vi "velocity control.vi"() -> ()   [LabVIEW 2018]
uses:
  <vilib>/Platform/TimedLoop/XDataNode/timing_clust.ctl
  <vilib>/Platform/TimedLoop/XDataNode/nitl_modes.ctl
  <vilib>/Platform/TimedLoop/XDataNode/wakeup.ctl
  <vilib>/FPGAPlugInAG/myRIO-1900/niLvFpga_Open_myRIO-1900.vi
  <vilib>/rvi/interface/common/dynamic/niFpgaDynamicAddResources.vi
  <vilib>/Utility/error.llb/Error Cluster From Error Code.vi
  <vilib>/rvi/errors/niLvFpgaAdjustHostInterfaceError.vi
  <vilib>/rvi/interface/nirviOpenFPGA/nirviOpenFPGA.xnode
  FPGA Bitfiles/Dentalrobot_FPGATarget_FPGADentalroboto_PTkoih3chUc.lvbitx
  FPGA/FPGA_myRIO.vi
  <vilib>/rvi/interface/nirviReadWriteControl/nirviReadWriteControl.xnode
  <vilib>/Platform/TimedLoop/XDataNode/XDataNode.xnode
  <vilib>/Platform/TimedLoop/XDataNode/XDNodeRunTimeDep.lvlib
  <vilib>/rvi/interface/Simulation/niFpgaSimulationCallBeginRW.vi
  NiFpgaLv.dll
panel:
  out "V' 2":dbl
  out "Waveform Chart 2":dbl(graph)
  out "Duty Cycle (Abs)":dbl
  in  "PID Gains":cluster{"Kp":dbl, "Kd":dbl, "Ki":dbl}={"Kp"=0.0021, "Kd"=0.0005, "Ki"=0.0005} {"Kp" step=0.001 format="%#_8f"; "Kd" step=0.01; "Ki" format="%#_6f"}
  out "V'":dbl
  in  "Desired Velocity":dbl step=10.0
  in  "Counts/revolution":i32=34304
  out "JumpBy2Error 4":i16
  out "Waveform Chart":dbl(graph)
  in  "stop":bool
  out "Position4":i32
  in  "Reset 4":bool
  in  "DIR4":bool
  in  "ENA4":bool
  out "finished late":dbl
  # "275:1   140800\n67:1      34304"
  # "rpm"
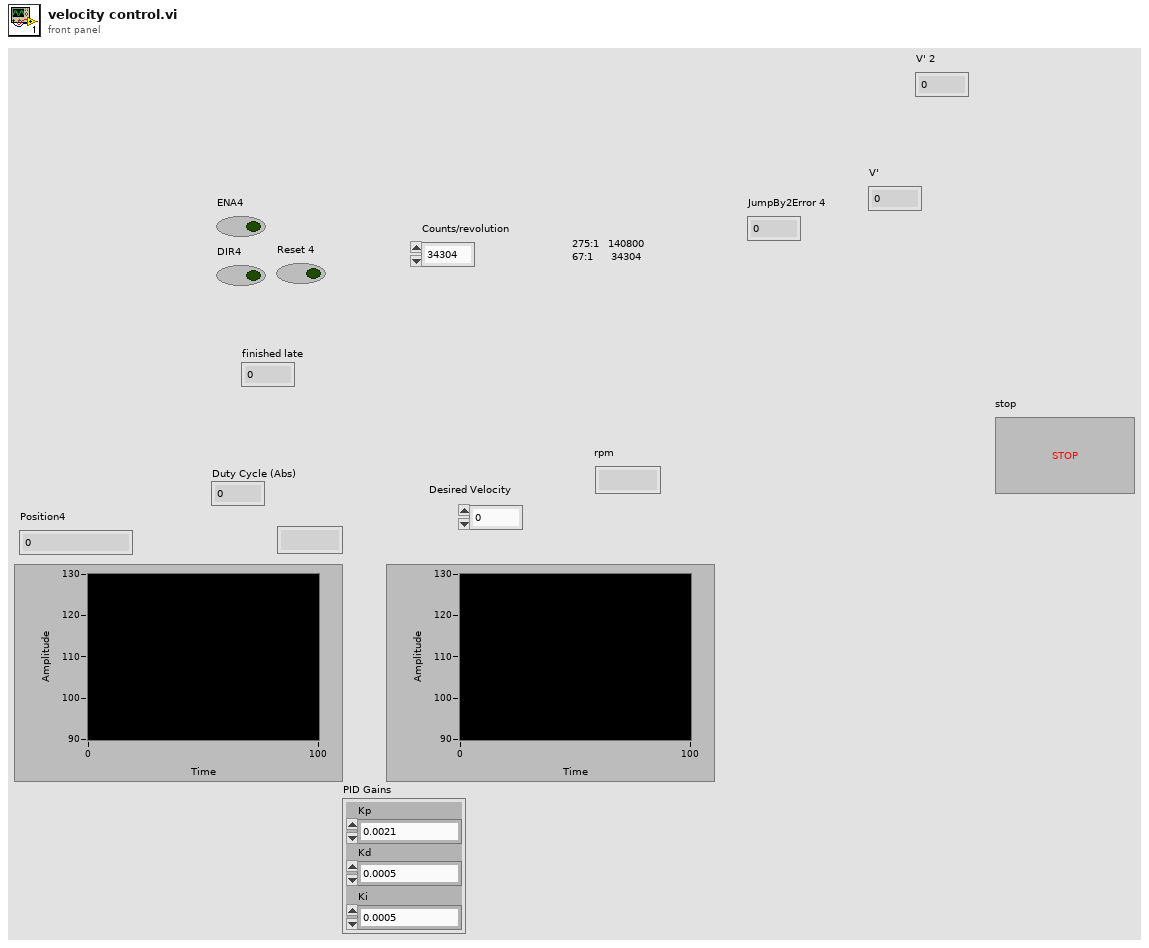
[diagram p1: front panel]
types:
  T1 = typedef "XDNodeRunTimeDep.lvlib/timing_clust.ctl" = cluster{"Expected End [f-1]":u64, "Actual End [f-1]":u64, "Finished Late? [f-1]":bool, "Expected End [i-1]":u64, "Actual End [i-1]":u64, "Finished Late? [i-1]":bool, "Expected Start [i]":u64, "Actual Start [i]":u64, "Expected Start [f]":u64, "Actual Start [f]":u64, "Source Name":string, "Structure Name":string, "Period":i64, "Deadline":i64, "Offset":i64, "Start":i64, "Priority":i32, "Timeout":i32, "Mode":T2, "Wakeup Reason":T3, "Error":errorcluster, "Source Type":string, "Secondary Source Type":string, "Global End Time":u64, "Global Start Time":u64, "Frame Duration":u64, "Iteration Duration":u64, "Assigned CPU":i32, "I/O Scan Engine Mode":u32}
  T2 = typedef "XDNodeRunTimeDep.lvlib/nitl_modes.ctl" = enum32{"No Change", "Process missed periods, maintain original phase", "Discard missed periods, maintain original phase", "Process missed periods, ignore original phase", "Discard missed periods, ignore original phase"}
  T3 = typedef "XDNodeRunTimeDep.lvlib/wakeup.ctl" = enum32{"Normal", "Aborted", "Asynchronous wakeup", "Timing source error", "Timed loop error", "Timeout"}
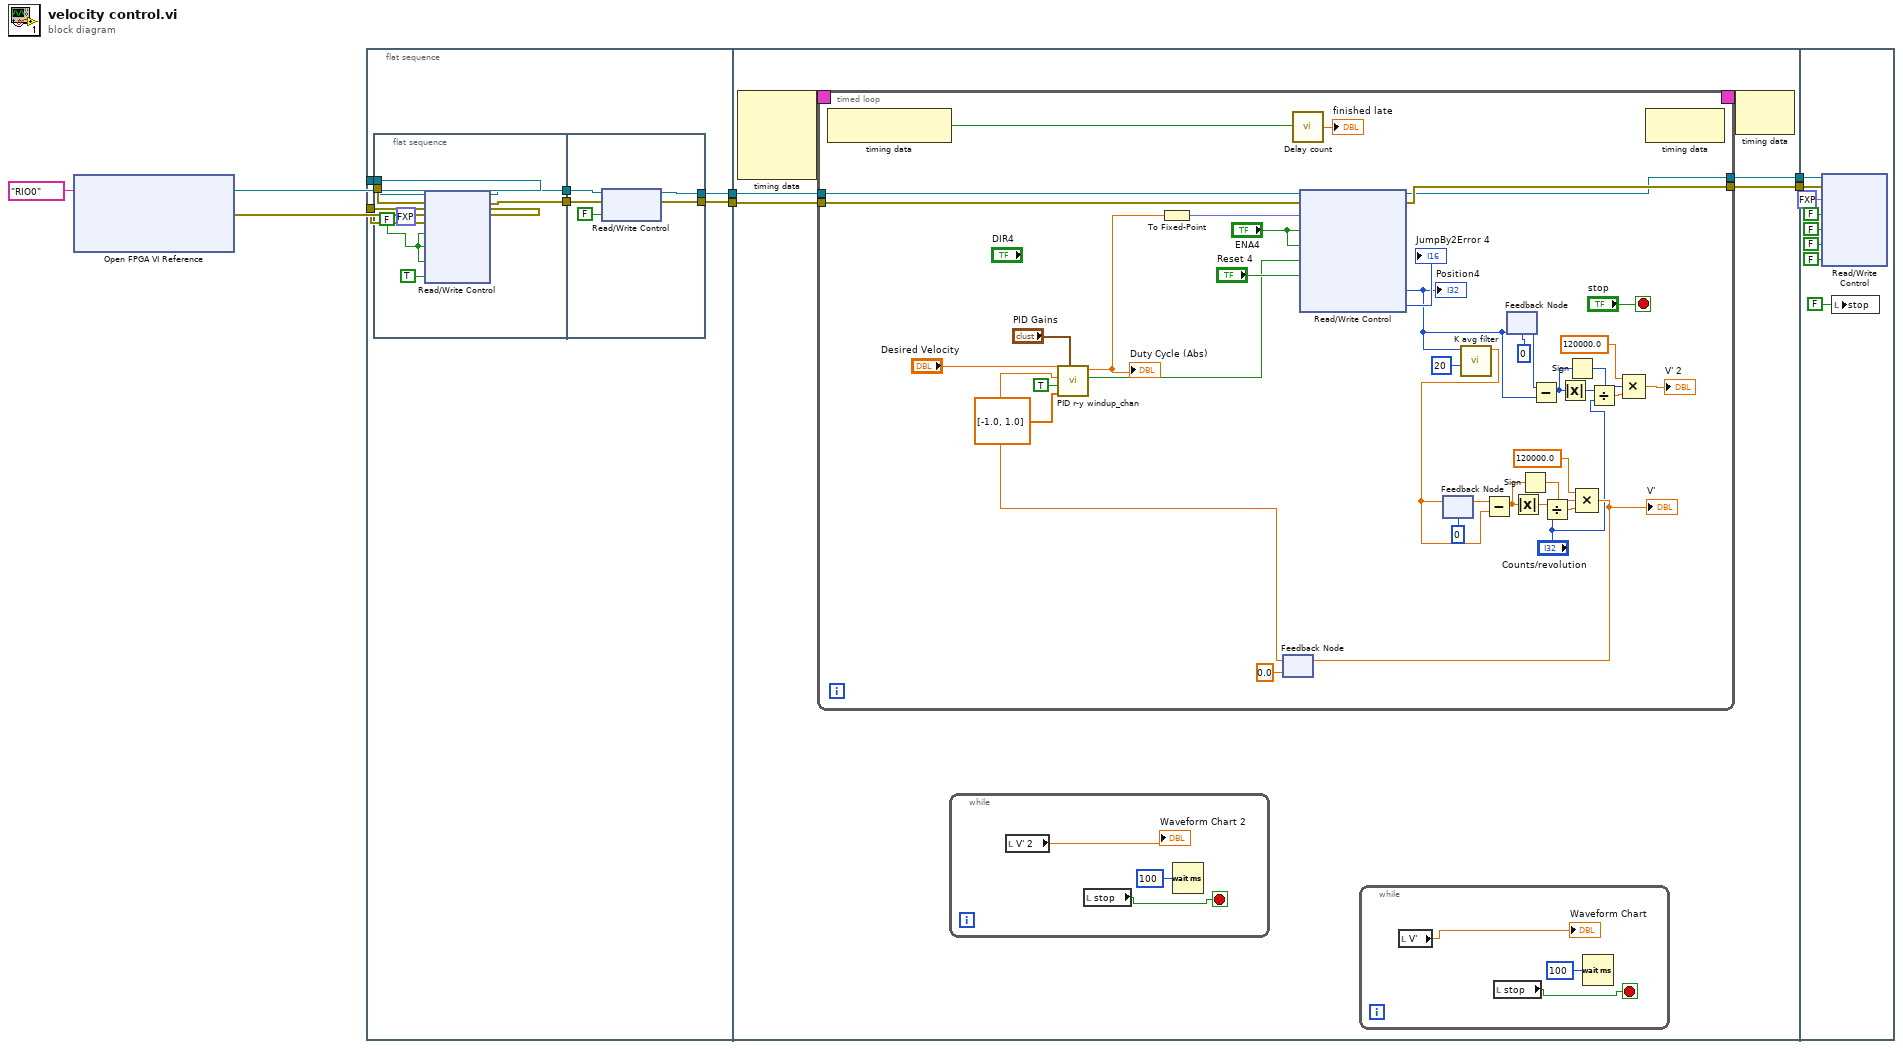
[diagram p0: block diagram]
diagram:
  n1 = xnode "Open FPGA VI Reference"("resource name"=tag "RIO0") -> ("FPGA VI Reference Out"=w3:refnum<k20>, "error out"=w2:errorcluster)  [unwired: 1 in]
  n2 = flat-sequence {
    tunnel: [w13] -> w7
    tunnel: [w8] -> w6
    tunnel: w3 -> [w12]
    tunnel: w2 -> [w11]
    tunnel: w7 -> [w26]
    tunnel: w6 -> [w27]
    tunnel: [w29] -> w5
    tunnel: [w28] -> w4
    tunnel: w5 -> [w89]
    tunnel: w4 -> [w88]
    frame #0 {
      n3 = flat-sequence {
        tunnel: w12 -> [w16]
        tunnel: w11 -> [w15]
        tunnel: [w18] -> w10
        tunnel: [w17] -> w9
        tunnel: [w23] -> w13
        tunnel: w10 -> [w24]
        tunnel: w9 -> [w25]
        tunnel: [w22] -> w8
        frame #0 {
          w20 = FALSE
          n4 = xnode "Read/Write Control"("FPGA VI Reference In"=w16, "error in"=w15, "CH4 DC"=fxp<+,32,0> 0.0, "ENA4"=w20, "STBY4"=w20, "DIR4"=w20, "Reset 4"=TRUE) -> ("FPGA VI Reference Out"=w18:refnum<k20>, "error out"=w17:errorcluster)
        }
        frame #1 {
          n5 = xnode "Read/Write Control"("FPGA VI Reference In"=w24, "error in"=w25, "Reset 4"=FALSE) -> ("FPGA VI Reference Out"=w23:refnum<k20>, "error out"=w22:errorcluster)
        }
      }
    }
    frame #1 {
      n6 = node-c288() -> (w31:T1)  [unwired: 4 in]
      n7 = timed-loop {
        timing: w31 -> [_]
        timing-out: [_] -> w30
        tunnel: w26 -> [w76]
        tunnel: w27 -> [w75]
        tunnel: [w67] -> w29
        tunnel: [w68] -> w28
        stop <- "stop" stop-if-true
        n8 = node-c288() -> (w74:bool)  [unwired: 1 in]
        n9 = feedback #1(0.0) -> (w50:dbl)
        n10 = call "PID r-y windup_chan.vi"("PID Gains"="PID Gains", "Saturation"=dbl[] [-1.0, 1.0], "Reverse Motor?"=TRUE, "Encoder position"=w50, "Reference"="Desired Velocity") -> ("DIR"=w60:bool, "Duty Cycle (Abs)"=w58:dbl)  [unwired: 3 in, 2 out]
        "Duty Cycle (Abs)" <- w58
        n11 = To Fixed-Point(number=w58) -> (fixed-point=w63:fxp<+/-,32,16>)  [unwired: 1 in]
        n12 = call "Delay count.vi"("Finished Late? [i-1]"=w74) -> ("Count"=→"finished late":dbl)
        n13 = xnode "Read/Write Control"("FPGA VI Reference In"=w76, "error in"=w75, "CH4 DC"=w63, "ENA4"="ENA4", "STBY4"="ENA4", "DIR4"=w60, "Reset 4"="Reset 4") -> ("FPGA VI Reference Out"=w67:refnum<k20>, "error out"=w68:errorcluster, "Position4"=w38:i32, "JumpBy2Error 4"=→"JumpBy2Error 4":i16)
        "Position4" <- w38
        n14 = feedback #2(0 ("Position4")) -> (w65:dbl)
        n15 = call "K avg filter.vi"("num avg"=20, "input"=w38) -> ("output"=w49:dbl)  [unwired: 9 in]
        n16 = feedback-in #2(w49) -> ()
        n17 = Subtract(x=w65, y=w49) -> (x-y=w53:dbl)
        n18 = feedback #3(0 ("Position4")) -> (w41:i32)
        n19 = feedback-in #3(w38) -> ()
        n20 = Absolute Value(x=w53) -> (abs(x)=w54:dbl)
        n21 = Sign(1:w53) -> (0:w52:dbl)
        n22 = Subtract(x=w41, y=w38) -> (x-y=w45:i32)
        n23 = Divide(x=w54, y="Counts/revolution") -> (x/y=w66:dbl)
        n24 = Absolute Value(x=w45) -> (abs(x)=w44:i32)
        n25 = Sign(1:w45) -> (0:w46:i32)
        n26 = Compound Arithmetic op=MULTIPLY(120000.0 ("x"), w52, w66) -> (w55:dbl)
        "V'" <- w55
        n27 = feedback-in #1(w55) -> ()
        n28 = Divide(x=w44, y="Counts/revolution") -> (x/y=w40:dbl)
        n29 = Compound Arithmetic op=MULTIPLY(120000.0 ("x"), w46, w40) -> (→"V' 2":dbl)
        n30 = node-c288() -> ()  [unwired: 1 in, 1 out]
      }
      n31 = while {
        stop <- w33 stop-if-true
        n32 = local read "V' 2"() -> (→"Waveform Chart 2":dbl)
        n33 = local read "stop"() -> (w33:bool)
        n34 = Wait (ms)(milliseconds to wait=u32 100) -> ()  [unwired: 1 out]
      }
      n35 = while {
        stop <- w36 stop-if-true
        n36 = local read "V'"() -> (→"Waveform Chart":dbl)
        n37 = local read "stop"() -> (w36:bool)
        n38 = Wait (ms)(milliseconds to wait=u32 100) -> ()  [unwired: 1 out]
      }
      n39 = node-c288(w30) -> ()  [unwired: 1 out]
    }
    frame #2 {
      n40 = xnode "Read/Write Control"("FPGA VI Reference In"=w89, "error in"=w88, "CH4 DC"=fxp<+,32,0> 0.0, "ENA4"=FALSE, "STBY4"=FALSE, "DIR4"=FALSE, "Reset 4"=FALSE) -> ()  [unwired: 2 out]
      n41 = local write "stop"(FALSE ("stop")) -> ()
    }
  }
